vi "lsl pull sample d.vi"(0 "in":cluster{}, 1 "ec":i32, 5 "buffer":dbl, 7 "buffer_elements":i32, 9 "timeout":dbl, 11 "error in (no error)":errorcluster) -> (3 "ec out":i32, 4 "in out":cluster{}, 6 "buffer out":dbl, 8 "function return":dbl, 15 "error out":errorcluster)   [LabVIEW 2018, in "liblsl-LabVIEW.lvlib"]
doc: "extern LIBLSL_C_API double lsl_pull_sample_d(lsl_inlet in, double *buffer, int32_t buffer_elements, double timeout, int32_t *ec);"
uses:
  <userlib>/liblsl-LabVIEW/liblsl-LabVIEW.lvlib
  <userlib>/liblsl-LabVIEW/liblsl64.dll
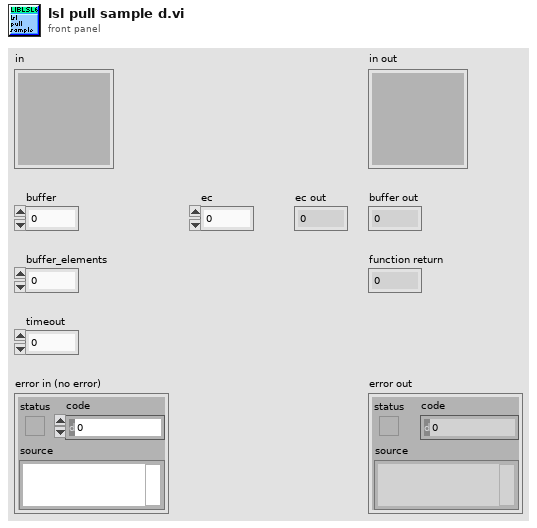
[diagram p1: front panel]
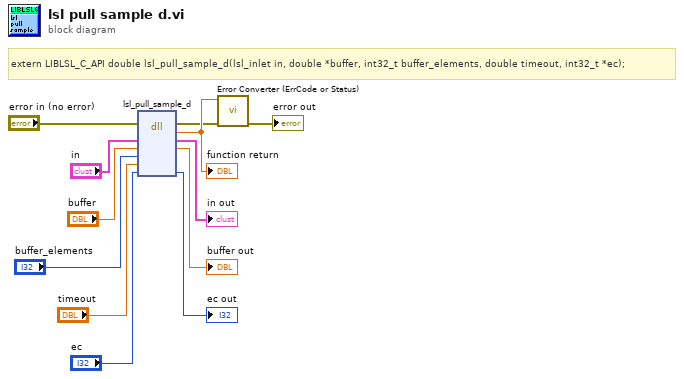
[diagram p0: block diagram]
diagram:
  # "extern LIBLSL_C_API double lsl_pull_sample_d(lsl_inlet in, double *buffer, int32_t buffer_elements, double timeout, int32_t *ec);"
  n1 = dll-call lib="C:/Program Files/National Instruments/LabVIEW 2018/user.lib/liblsl-LabVIEW/liblsl64.*" fn="lsl_pull_sample_d"(error in="error in (no error)", "in"="in", "buffer"="buffer", "buffer_elements"="buffer_elements", "timeout"="timeout", "ec"="ec") -> (error out=w2:errorcluster, w12:dbl, "in"=→"in out":cluster{}, "buffer"=→"buffer out":dbl, "ec"=→"ec out":i32)  [unwired: 4 in, 1 out]
  "function return" <- w12
  n2 = call <userlib>:"Error Converter (ErrCode or Status).vi"("error in (no error)"=w2, "error code"=w12) -> ("error out"=→"error out":errorcluster)  [unwired: 9 in]
